vi "UHR-Fleezers Control (host) -Leonardo 04-2018 V4_fish.vi"(0 "Tab Green FB":T5(tab)=enum."Trap Control (RF)") -> ()   [LabVIEW 2014] (continued)
0.042672538888036585, 0.042644759345288163, 0.04261697980253975, 0.04258920025979133, 0.04256142071704291, 0.04253364117429449, 0.04250586163154607, 0.04247808208879765, 0.04245030254604923, 0.04242252300330081, 0.042394743460552387, 0.04236696391780398, 0.04233918437505556, 0.04231140483230714, 0.042283625289558716, 0.042255845746810294, 0.04222806620406188, 0.04220028666131346, 0.04217250711856504, 0.042144727575816616, 0.0421169480330682, 0.04208916849031978, 0.04206138894757136, 0.04203360940482294, 0.04200582986207452, 0.0419780503193261, 0.041950270776577675, 0.04192249123382926, 0.041894711691080846, 0.041866932148332425, 0.041839152605584004, 0.04181137306283558, 0.04178359352008716, 0.04175581397733874, 0.04172803443459032, 0.0417002548918419, 0.04167247534909349, 0.04164469580634507, 0.04161691626359665, 0.04158913672084823, 0.041561357178099806, 0.0415335776353514, 0.04150579809260298, 0.041478018549854556, 0.041450239007106135, 0.041422459464357714, 0.04139467992160929, 0.04136690037886087, 0.04133912083611246, 0.04131134129336403, 0.04128356175061562, 0.04125578220786719, 0.04122800266511878, 0.04120022312237036, 0.04117244357962194, 0.041144664036873516, 0.041116884494125094, 0.04108910495137668, 0.04106132540862826, 0.04103354586587984, 0.041005766323131417, 0.040977986780383, 0.04095020723763458, 0.04092242769488616, 0.04089464815213774, 0.04086686860938932, 0.0408390890666409, 0.04081130952389249, 0.04078352998114407, 0.040755750438395646, 0.040727970895647225, 0.040700191352898804, 0.04067241181015039, 0.040644632267401976, 0.04061685272465355, 0.04058907318190513, 0.04056129363915671, 0.04053351409640829, 0.04050573455365987, 0.04047795501091145, 0.040450175468163034, 0.04042239592541461, 0.0403946163826662, 0.04036683683991778, 0.04033905729716935, 0.040311277754420935, 0.040283498211672514, 0.0402557186689241, 0.04022793912617567, 0.04020015958342725, 0.040172380040678836, 0.04014460049793042, 0.040116820955182, 0.04008904141243358, 0.04006126186968516, 0.04003348232693674, 0.04000570278418832, 0.03997792324143991, 0.03995014369869149, 0.039922364155943066, 0.039894584613194645, 0.03986680507044622, 0.0398390255276978, 0.03981124598494939, 0.03978346644220096, 0.039755686899452546]
  in  "Tab APD Timing":enum32{"Timing", "MCL Scan", "Analog Out"}(tab)=enum."MCL Scan"
  out "APD 2 Gate Late Counter":u32
  out "APD 2 Gate Relative Phase":i16
  in  "Phase Adj. (APD 2 Gate)":i16=20
  in  "Initial Phase Adjustment (APD 2 Gate)":i16=45
  out "APD 1 Gate Late Counter":u32
  in  "- phase (APD 1 Gate)":bool
  in  "+ phase (APD 1 Gate)":bool
  out "APD 1 Gate Relative Phase":i16
  in  "Phase Adj. (APD 1 Gate)":i16=20
  in  "Initial Phase Adjustment (APD 1 Gate)":i16=50
  in  "Save APD Data\nwith Trap Data":bool=TRUE
  out "APD FIFO Elements Remaining":u32
  in  "- phase (APD Acq)":bool
  in  "+ phase (APD Acq)":bool
  out "APD Acq Late Counter":u32
  out "APD Acq Relative Phase":i16
  in  "Phase Adj. (APD Acq)":i16=20
  in  "Initial Phase Adjustment (APD Acq)":i16
  in  "Invert APD Gate":bool caption="Invert Gate"
  in  "APD Gate OFF Count":u32=450 caption="Gate OFF Count"
  in  "APD Gate ON Count":u32=150 caption="Gate ON Count"
  in  "APD Gate":enum32{"ON", "OFF", "Interlace"}(radio)=enum."Interlace"
  in  "APD Integration Time (s)":dbl=0.01 caption="Integration Time (s)"
  out "APD Acq Rate (Hz)":dbl=100.0 caption="Rate (Hz)"
  out "APD Samples/FIFO Acq.":dbl=30.0
  out "APD Elements/DMA read":u32=60
  out "APD Int. Count":u32=400000 format="%.0p"
  in  "+ phase (APD 2 Gate)":bool
  in  "- phase (APD 2 Gate)":bool
  in  "APD FIFO Depth (requires restart)":u32=300000 format="%.0p"
  in  "Tab MCL Misc":enum32{"PSD X", "PSD Y", "Other Data Channel"}(tab)
  out "Data map":dbl[][](graph)=[[-0.01671932143166878, -0.016392818706373227, -0.016060241502617766, -0.016885058281480972, -0.016633639866051188, -0.01614297111485056, -0.01624632439809061, -0.016223291898502697, -0.016322135358181895, -0.015998827366942206, -0.01674383457317074, -0.016349622303473588, -0.01611571290004051, -0.015972334649942688, -0.016306900004507047, -0.016265804263496074, -0.0160006281874421, -0.01579815848604542, -0.015557994770877373, -0.01623934207097493], [-0.016401746716030643, -0.016486228679580477, -0.016405819418185925, -0.017006941359896506, -0.01609698301441303, -0.0159938373980257, -0.015449969664593804, -0.016068061784641922, -0.016115383931390913, -0.015648222289449794, -0.01653040435156989, -0.01664368093936457, -0.015976629115606142, -0.015769041987412753, -0.015716784490458328, -0.016104708313091028, -0.015807740113897233, -0.016007795937736217, -0.015716865824611653, -0.016131560547170874], [-0.016881180243279052, -0.016682362901092443, -0.01653521208533211, -0.016569663649832547, -0.016584350108926265, -0.015788034358096, -0.01572997381191265, -0.016848256863673278, -0.016450971094654886, -0.016646544202256155, -0.016533647976865372, -0.01643411945121718, -0.01642968729491641, -0.015287525792493872, -0.015664412933211656, -0.016705160893495323, -0.01634751515697455, -0.016385950364931786, -0.01641611962972788, -0.016336369365154098], [-0.016944386833653874, -0.017209095062396696, -0.01643647162326984, -0.0169434622427136, -0.01645749558522405, -0.016283892481898044, -0.016603972603686925, -0.016019804038190342, -0.01633990863890397, -0.016779562572954584, -0.01649257003377154, -0.01633196294664365, -0.01681717360495772, -0.016151141680784836, -0.015631110690343758, -0.01616762209708058, -0.01570812545409377, -0.016238042109499973, -0.016140009377557954, -0.015480352129179791], [-0.016627380272623872, -0.016987040432100503, -0.0162998105424607, -0.01635693474229572, -0.016728613514399027, -0.015877063835195653, -0.01632422175035657, -0.015987062444069455, -0.016082210905250194, -0.016795453503208664, -0.0170165982501747, -0.016041147401410074, -0.015844635002206515, -0.01588368721722097, -0.016415515701510675, -0.01625686223052733, -0.015522307984761095, -0.016125254990784654, -0.016133227363549094, -0.016093654313254407], [-0.016918226627058684, -0.016546339201955095, -0.016238630263811032, -0.01698719582491472, -0.016111760237599002, -0.016169388046078873, -0.01635628471807927, -0.016477982760217016, -0.016022494806163096, -0.01635452184408291, -0.016437829589091835, -0.01620151587720066, -0.016192846971583803, -0.016361330735626047, -0.015920360440429684, -0.015596058601637491, -0.015839057608204695, -0.01590683226225114, -0.016147455226815495, -0.016061133185195295], [-0.016634948322751798, -0.016569012123295146, -0.01662465918442623, -0.01677966319575081, -0.016244237674368125, -0.016934028324529424, -0.015994902143504568, -0.01577806108898649, -0.015702882269567658, -0.01637426003303808, -0.016516796952512437, -0.01646180977161214, -0.017050841082784957, -0.015210920961454804, -0.016180578875882937, -0.01607665952058283, -0.01643056573904152, -0.01624726697921726, -0.016811320756287537, -0.015704237088347145], [-0.016797771368752906, -0.01616083928333069, -0.016453251971550422, -0.01638112181272177, -0.01590261356594244, -0.01608147749759244, -0.016020370516697566, -0.01666407664114518, -0.01638481284701757, -0.016175328500489604, -0.015634096607040564, -0.01659680945708638, -0.01626086024191585, -0.016096523812787963, -0.015760521307245458, -0.01615157630765101, -0.01563169067138887, -0.016252628883934674, -0.016238504839935688, -0.016296984466382107], [-0.01667963634531472, -0.015869270181190567, -0.01639782773103042, -0.01636439382881424, -0.01666285543553242, -0.016692875783958446, -0.016121724588237546, -0.016079967645743654, -0.01632967716613466, -0.0165840590606689, -0.01625421166976198, -0.016098422085292646, -0.016839026057991122, -0.01618499247497865, -0.015391600029151147, -0.016339655626827314, -0.015612166346566772, -0.015935379715422582, -0.015751812989013417, -0.016043659821299468], [-0.016548348623009697, -0.016991017407413864, -0.016507403110123067, -0.016536793878207376, -0.016691120016137963, -0.01577327808799238, -0.016241167864690632, -0.016068735698142586, -0.015840387814149363, -0.016134357225980472, -0.015841333026290365, -0.0163038114660657, -0.01664004009343323, -0.015517995684912076, -0.01510255011893393, -0.016011490555515644, -0.01579492187645071, -0.016061693314939115, -0.016070791499276448, -0.015958266458419586], [-0.017158052821315092, -0.016990745992594425, -0.01659770916824297, -0.016038631482428484, -0.016146804022232154, -0.01576224906436341, -0.016188682344964726, -0.016682643876198163, -0.016363274145684666, -0.01639850086318443, -0.015896821220835786, -0.015725853678146523, -0.01601090474694708, -0.015561700057052, -0.015999978841264924, -0.01601836056022779, -0.016765653382201824, -0.016096916088969352, -0.016073837821775124, -0.015692878955540758], [-0.01663419671959083, -0.016709422884628247, -0.017440867448447667, -0.016794212435564802, -0.016747490720603195, -0.017381751349696366, -0.016447004176656708, -0.016200072448833015, -0.016045160782039845, -0.01632124390318996, -0.01679169430451878, -0.016160654157203025, -0.016749084172300182, -0.015317451826774697, -0.01616958983467165, -0.015522373654827837, -0.016042029406509332, -0.016273918604509642, -0.016417636335760946, -0.01644358854973573], [-0.016334373306253872, -0.016757773312361682, -0.016379901767213538, -0.016648254461466998, -0.016415141976627915, -0.016163802224577726, -0.01585938187523836, -0.01585373106879133, -0.015975877635193418, -0.01599748687305492, -0.016737850820893803, -0.01594503246026053, -0.01605934628998727, -0.0158171814426758, -0.015143820145612868, -0.016535815039113604, -0.01611350163485256, -0.01603586147994221, -0.016191023597649318, -0.015673182413705102], [-0.016700857633048308, -0.017051706885756718, -0.016395162126784154, -0.016864165985049667, -0.01667278712452, -0.016023236569300325, -0.015936447644162688, -0.01626053315184134, -0.016666644977778797, -0.01651990276982608, -0.01690611112853018, -0.016570014742366936, -0.016014494913507715, -0.016334286074074115, -0.01621235686701924, -0.01653022812336152, -0.01583634924223019, -0.016281303974484927, -0.01653990312391212, -0.015384206653677268], [-0.016471441301573585, -0.01647096314202187, -0.016715886966535524, -0.015878302888681167, -0.016818970876684446, -0.016713152489800882, -0.0154648252478201, -0.016328530500277577, -0.015836781582585016, -0.01591923201699931, -0.016315094505816256, -0.015951841421804724, -0.01608430179945204, -0.015957272458344565, -0.015751249520465478, -0.016350306857141315, -0.015517909552404317, -0.015884662571158274, -0.016211720964471307, -0.01537858018482844], [-0.01674440523726064, -0.016870567772511377, -0.016213148874409115, -0.016888734754126403, -0.017090609693170035, -0.01659256562080198, -0.01625635717081822, -0.016107107745803876, -0.016234190134722645, -0.016577197956586683, -0.01658670958631228, -0.016563728816596346, -0.016688515093891267, -0.016736196160361996, -0.015994597797780702, -0.016061666241292242, -0.015206770358209283, -0.01656914278587982, -0.01606315534154764, -0.015681866815853374], [-0.016944331036564515, -0.017205260427342613, -0.01677120483170293, -0.016402843466637763, -0.01674116281665193, -0.016423395631415146, -0.01525500299962603, -0.01627542397053335, -0.016664853908603776, -0.01620332976021642, -0.015950564835878013, -0.01610107356411497, -0.016396683154864377, -0.015976631236977498, -0.015478300298060717, -0.015835627632208554, -0.01604600189786053, -0.015850180758366084, -0.01603596051783181, -0.015769623989901102], [-0.016857923835780924, -0.016573198672727902, -0.016660307411618773, -0.016198760579099178, -0.016151481374992453, -0.01623511193332007, -0.015818969815924802, -0.01644510963983431, -0.015972042272190907, -0.01666642359581892, -0.01666443700190194, -0.016438254918363447, -0.016138118663893655, -0.015691974269895034, -0.016587077315345165, -0.015965118060360686, -0.015699839910512218, -0.01561194620613338, -0.016186792034230305, -0.016197922335520733], [-0.016756662992071368, -0.017021980605505502, -0.01671540550240299, -0.016161860765568574, -0.016256637402529132, -0.01604906368842445, -0.016092507257301394, -0.01617438393323743, -0.016105543848009572, -0.016246592326198385, -0.016142744624025374, -0.016159689527728567, -0.016177575339496836, -0.015961391152738445, -0.015789242903564853, -0.016290502978789936, -0.01590902706214275, -0.016035878036151207, -0.0163699057102928, -0.016166856731619543], [-0.016230743921604517, -0.01699457586491366, -0.01691575006710251, -0.01691567874763252, -0.016632348348462205, -0.01564006866069024, -0.015669555325846102, -0.01675726036853814, -0.015659388136628594, -0.01633203630678029, -0.016275904140963263, -0.01599466989252362, -0.01670183436780044, -0.016544315654085533, -0.015882735536646285, -0.01634814491721433, -0.015693511174422668, -0.015857069610244905, -0.015293298228102974, -0.01570879180052374], [-0.016746550537387085, -0.016635756849929545, -0.01704192789682773, -0.01592942336549498, -0.016565335498658518, -0.016559981627150607, -0.016370390094235444, -0.016204117687222342, -0.01636993721064581, -0.016019023809705737, -0.01624713908528634, -0.01653713290533686, -0.01654191191022731, -0.015871787270804183, -0.016600435605206076, -0.016053794928515903, -0.015786397557799592, -0.016167422435048453, -0.016149009764007245, -0.015779827376486453], [-0.017141787830569893, -0.01685604196926299, -0.016770676218784503, -0.01657265724540346, -0.016973351148096293, -0.016347677914333066, -0.015700463473615457, -0.0157292679709582, -0.016282549721629708, -0.015799962485816943, -0.0169651499113691, -0.017005390716294616, -0.01616841590634147, -0.01579805772887789, -0.015884669429112312, -0.01687947774540062, -0.015546104827296667, -0.01606408203496036, -0.015764690031214893, -0.016077969368821936], [-0.01755128513645066, -0.016614441354853425, -0.01642295621649906, -0.016572002735089818, -0.016539344978417192, -0.01665672671509038, -0.01610564101766388, -0.0167710479608722, -0.01604147346071364, -0.015915051759660022, -0.01690954942974296, -0.01618215110656205, -0.01687103577661275, -0.015704550539293104, -0.01567934362211993, -0.015968805810754147, -0.01586985536309292, -0.015848872001954256, -0.015923479964089694, -0.015604572794266433], [-0.01700702905775247, -0.016405242404623068, -0.016957584669743626, -0.01649808356316003, -0.015831866505709048, -0.01650461850371917, -0.015987113078007254, -0.015834023912635466, -0.015505062044615166, -0.016233666617861173, -0.016028249584376462, -0.016292798595496677, -0.016811560188299345, -0.015802581883183398, -0.015195148613460024, -0.015765465657774175, -0.016294889918615045, -0.01647530657977607, -0.016354233471026363, -0.01618598563271133], [-0.016283357847285636, -0.01655641981831666, -0.016127059444156554, -0.016293855360523378, -0.01631947219897442, -0.016398508430939616, -0.0164960599809452, -0.01635229032278839, -0.016150072161158744, -0.01646190473964058, -0.016283962555137702, -0.01689040784367708, -0.016767163139998632, -0.016438000493173108, -0.015954956500429416, -0.016569056147695202, -0.016605504963760735, -0.015329313107534112, -0.01578842030659742, -0.015421959499234628], [-0.016479987599589248, -0.01644678482494596, -0.016512996052180717, -0.01623094473834884, -0.016604746810030113, -0.016230213519226107, -0.016359208382350467, -0.01609761921903255, -0.016464485575532387, -0.015985272322973462, -0.015774520381458212, -0.01632178510310122, -0.016823351362691343, -0.01643553466150876, -0.015434648968053383, -0.01640702032901096, -0.015639626970513753, -0.01608966370811705, -0.016018362361111357, -0.01607982188546427], [-0.016959739645157706, -0.016680901866661726, -0.015836205448559966, -0.016650560318028734, -0.015979362423611275, -0.015641297610719303, -0.015788746501915876, -0.016033508703118756, -0.01595573902096323, -0.016363948579213562, -0.016349864006002027, -0.016495398899173445, -0.016242648234899834, -0.016920033344786076, -0.016276181128461735, -0.016473741446416813, -0.015963577017676644, -0.015565621002678179, -0.01634988477510272, -0.016759987490697584], [-0.016465195958807775, -0.016666490625723715, -0.016658908615375, -0.01597417902764041, -0.016394946754303752, -0.016153528909152313, -0.016275277887248356, -0.016575820504070977, -0.016165440248126276, -0.0158334592734765, -0.016393067206609387, -0.016885479811953534, -0.016471593134372298, -0.017124297138208497, -0.01548599428740715, -0.016309544928836586, -0.015739577267293366, -0.016315386973421362, -0.016361118135948566, -0.016635949477566882], [-0.016680470580762462, -0.016967020008211, -0.017070403001069857, -0.015793158201855152, -0.01661718510493328, -0.01621301409151063, -0.015497330917384148, -0.016267684516616924, -0.015545683307124036, -0.01584462817622427, -0.016830529260392843, -0.016203294725707643, -0.016943290418910587, -0.015581438668509352, -0.015578492450734066, -0.01643368853494311, -0.016285119780950222, -0.015912568651561352, -0.015719368411857025, -0.015732642681635923], [-0.017056323385982973, -0.017071971641855074, -0.01624203196673346, -0.016577086084052214, -0.016198385464505236, -0.015959998936922397, -0.015388246890736087, -0.01690871560472578, -0.016520770777269024, -0.016719342780151844, -0.01589885976225658, -0.016316317143634285, -0.015927259253864068, -0.01613903479860508, -0.015938319643326725, -0.015996730877187566, -0.01552190097834432, -0.016279927776335308, -0.015995176436170485, -0.015804091652970826], [-0.017190435316337342, -0.016575163169333516, -0.01629659819256952, -0.016774256975583077, -0.015978440181354282, -0.016162892801179076, -0.01620143768882657, -0.016215940324925678, -0.016085616640623322, -0.01624795446292185, -0.015590279490139558, -0.016351775677783426, -0.01628162630120476, -0.016736583715483217, -0.015290607493835316, -0.01675006130238602, -0.016112399997689694, -0.016085396155956493, -0.01584495781031281, -0.016031709625742012], [-0.017226310157841672, -0.0164663033859778, -0.01638852606295136, -0.01642215259901681, -0.016566243818266997, -0.016484045986143257, -0.016452209817223822, -0.016464707609223313, -0.01598467645947642, -0.016476401570535384, -0.015529223129381136, -0.016802343788985992, -0.016417294815804, -0.016305476633183012, -0.015407470515554668, -0.01588918182788552, -0.015839354895906106, -0.016859219988342257, -0.016188952756112908, -0.015382351679335257], [-0.017044276140355946, -0.016525294382434108, -0.01600036800318285, -0.01692841042125611, -0.016063543400203904, -0.0167008216867912, -0.01583944304325613, -0.015982843969462788, -0.01610446772754332, -0.01650934416727942, -0.016660683575282727, -0.016326108469991264, -0.01614299940648814, -0.016050548764700443, -0.016131072933532012, -0.016315196635999143, -0.016225473554238007, -0.01551847935196565, -0.015874550726858914, -0.01566897000262655], [-0.016174756903461544, -0.01692999553661901, -0.01705167048362926, -0.01660949009366751, -0.016107419352032235, -0.016188509519945497, -0.015585853922651487, -0.01612262091090234, -0.016426426055949322, -0.01609822137272688, -0.016735004284984756, -0.016043599908818165, -0.016651804571551146, -0.01556136051538674, -0.015408827232157843, -0.015855874683892428, -0.015887023972496795, -0.01599811437353065, -0.015655637769778918, -0.015893480415302176], [-0.016396467105890343, -0.01690556505247584, -0.0163054855200399, -0.016446662941364928, -0.01622691165873451, -0.016690239637868323, -0.015785441074554568, -0.016620593981308673, -0.015765446409343138, -0.016270811628848948, -0.016094841434208293, -0.01632812303243944, -0.01619217328151394, -0.015836234359203484, -0.016074598803568225, -0.01532030760600064, -0.01657169575010852, -0.016393493124135967, -0.01597552762388542, -0.015565046037824628], [-0.016299520764774443, -0.016637551393085426, -0.016299287907039765, -0.01610813956937386, -0.016305200311999217, -0.016601228593523636, -0.016288899767132464, -0.016305235511310533, -0.016063090550620947, -0.01683118193989227, -0.015518909238992087, -0.01620458965118359, -0.01645647074542291, -0.015677575909554008, -0.015332584749786342, -0.016079840062543812, -0.016278322310175185, -0.01605786016548567, -0.01657700147769983, -0.01606751816440997], [-0.016441387384698882, -0.017325914631361444, -0.017225293509456174, -0.016118796157285526, -0.016362377734664042, -0.01516634537172325, -0.01608508664570788, -0.01572299536201756, -0.01616493137153105, -0.01621315960010322, -0.016750280429064943, -0.016228195768808316, -0.01653543568323192, -0.01645026349483051, -0.016050647149129828, -0.01642593239180811, -0.0161192309302286, -0.01629438826737352, -0.015557310160813994, -0.016021567325025916], [-0.01686693458295582, -0.016740786564424494, -0.01648453245605215, -0.01640092243822592, -0.01555424864442638, -0.01667099748425638, -0.016069415470156286, -0.01638225749592203, -0.01607630099787768, -0.01614344420814296, -0.016216929728619375, -0.016309670684273796, -0.015741358140653132, -0.015770999475234804, -0.01601963602183988, -0.01615265943136728, -0.016152653946118384, -0.01698528285009184, -0.015969420465915152, -0.01578449323306024], [-0.01598619419452168, -0.016362732490235912, -0.016433844312774552, -0.016357999277320685, -0.015969441982301692, -0.01621147526376268, -0.016085473373391473, -0.016306341052304336, -0.015855664982231947, -0.015900633884010838, -0.016902356755211914, -0.016434765274207237, -0.016180164153866673, -0.015973977144992546, -0.01589274164800459, -0.01640268056199417, -0.016415161422386984, -0.01617112040367598, -0.016354725082739732, -0.016206639631885546], [-0.016048964224847716, -0.016745007333129024, -0.017180534108641177, -0.016329775174222558, -0.016582289070660373, -0.016075138720435006, -0.016345162602564738, -0.016090296577092385, -0.016153752753705675, -0.016379459268123033, -0.016228628993078524, -0.016712275509199688, -0.015795168051192618, -0.015386431874568587, -0.01610093851445945, -0.01633598707495066, -0.015921284689633122, -0.016330315102764423, -0.015994974665173196, -0.015537812293197398]]
  in  "Channel":i32=4
  in  "Abort MCL Scan":bool
  out "MCL Scan I":u64=2
  out "MCL Scanning":bool
  in  "Start MCL Scan":bool
  out "wait to reset values":bool
  in  "Tab MCL Scan Settings":enum32{"Scan Settings", "MCL FPGA Loop Timing"}(tab)
  out "Total Time (s)":dbl=48.0
  in  "Scan lines (y)":u64=20
  in  "Fast Scan Dir":bool=TRUE
  in  "2D or 1D Scan":bool=TRUE
  out "Initial X":dbl=1.6310662274449115
  out "Initial Y":dbl=2.5691326639606933
  out "Time/f+b scan (s) (MCL)":dbl=2.4 caption="Time/scan (s)"
  in  "Number of scans (MCL)":u64=1 caption="Scans"
  in  "Scan steps (MCL)":u64=40 caption="Scan steps (x)"
  in  "N APD Samp/step":dbl=3.0
  in  "Scan Range (V)\n(of steps)":dbl=3.5
  in  "Restart DMA? (MCL)":bool=TRUE caption="Restart DMA?"
  in  "Continuous MCL Scanning":bool caption="Cont. Scanning"
  in  "Center Scan":bool=TRUE
  in  "Save Data (MCL)":bool=TRUE caption="Save Data"
  out "Actual Incr. int (MCL)":i16=462 caption="Incr. int"
  out "Desired incr (int)":dbl=462.098717948718
  out "Desired Scan Incr (V)":dbl=0.14102564102564102
  out "N sets should be saved (MCL)":dbl=160.0 caption="N sets should be saved"
  out "Data points/scans (MCL)":dbl=4800.0 caption="Data points/scans"
  out "Data points/scan (f+b)":dbl=240.0 caption="points/scan (f+b)"
  out "Cycles/step (MCL)":u64=2000 caption="Cycles/step" format="%.0p"
  out "Actual MCL Inc (V)":dbl=0.14099551377910702
  in  "Phase adjust (MCL)":i16 caption="Phase adjust"
  out "Relative Phase (MCL)":i16 caption="Relative Phase"
  in  "Initial Phase Adj. (MCL)":i16 caption="Initial Phase Adj."
  in  "Update Count (MCL)":u32=600
  in  "+ phase (MCL)":bool
  in  "- phase (MCL)":bool
  out "MCL Late Counter":u32
  in  "APD 1 AO Mult.":i16=1 min=1
  in  "APD 2 AO Mult.":i16=1 min=1
  in  "Tab Control 7":enum32{"Green FB Signals", "Slow MCL Scan"}(tab)
  out "Green FB Plot":dbl(graph)=-10.00030518509476
  out "MCL Scan 2":cluster{"Begin (V)":dbl, dbl, dbl[]}(graph)
  out "MCL Scan":cluster{"Begin (V)":dbl, dbl, dbl[]}(graph)
  in  "GI Frequency, ON count":u32=150 min=1 step=1
  in  "Invert GI":bool
  out "GI Late Counter":u32
  in  "Phase adj. (GI)":i16=5
  out "GI relative phase":i16
  in  "+ phase (GI)":bool
  in  "Initial Phase Adjustment (GI)":i16=4
  in  "GI Frequency, OFF count":u32=450 min=1 step=1
  in  "- phase (GI)":bool
  out "Green FB Signals (V)":cluster{"Y":dbl, "X":dbl, "Sum":dbl}={"Y"=-0.999969482421875, "X"=1.0, "Sum"=-10.00030518509476}
  out "Relative phase (Green FB)":i16
  in  "+ phase (Green FB)":bool
  in  "- phase (Green FB)":bool
  in  "Green FB Count":u32=600
  in  "Phase adj. (Green FB)":i16=10
  in  "Initial Phase Adjustment (Green FB)":i16=50
  in  "Green FB On/Off":bool
  in  "Green int current ON count adj":u32=150
  in  "Green FB Gains":T10={"proportional gain (Kc)"=10, "integral gain (Kc*Ts/Ti)"=5, "derivative gain (Kc*Td/Ts)"=0}
  in  "Green FB Setpoint (mV)":dbl=100.0
  in  "- phase (GI) 2":bool
  in  "Initial Phase Adjustment (GI) 2":i16=-100
  in  "+ phase (GI) 2":bool
  out "GI relative phase 2":i16
  in  "Phase adj. (GI) 2":i16=20
  out "GI Late Counter 2":u32
  in  "Negate X signals":bool
  in  "Trap Position FIFO Depth":u32=300000 format="%.0p"
  in  "# Samples/trap":u32=20000 format="%.0p"
  out "Trap AI Elements/DMA read":u32=320000 format="%.0p"
  out "Ave. Rate (Hz)":dbl=200000.0 format="%#_6p"
  out "Trap AI FIFO El. Rem.":u32 format="%.0p"
  in  "Phase adj. (AI1)":i16
  out "Relative phase (AI1)":i16
  in  "+ phase (AI1)":bool
  in  "- phase (AI1)":bool
  out "Late Counter (AI1)":u32
  in  "Initial Phase Adjustment (AI1)":i16=185
  out "AI rate (Hz)":dbl=200000.0 format="%#_6p"
  in  "AI Count (ticks)":u32=200
  out "# Samples/channel":u32=40000 format="%.0p"
  in  "Trap AI FIFO Depth":u32=340000 format="%.0p"
  in  "Detector Type":string(combo)="UCB Fleezers 052511"
  in  "N Acq Sets (Traps + Fl.)":i16=3
  in  "Sets to FIFO (Traps)":T15={"Set 1"=TRUE, "Set 2"=TRUE, "Set 3"=FALSE}
  in  "FPGA Ave.":dbl=1.0 min=1.0 step=1.0
  out "Ave. Period (s)":dbl=5e-06 format="%#_6p"
  out "DMA Update Period (s)":dbl=0.3
  out "FPGA Averaging":bool
  out "Trap Sets":u32=2
  out "Counts/DMA":dbl=12000000.0 format="%#_6p"
  out "Trap Pos FIFO El Remaining":u32=171
  out "Trap Pos Elements/DMA read":u32=120000 format="%.0p"
  out "Trap AI FIFO Timeout":u16
  out "Trap Pos FIFO Timeout":u16
  out "Waveform Chart":i32(graph)=320000
  out "error out 2":errorcluster
  in  "Lost Tether Alarm Threshold (pN)":dbl=0.5
  in  "AOM X Cal (nm/MHz)":dbl=160.0
  in  "MCL X Cal (nm/V)":dbl=1174.0
  out "X RF Amplitude Limits (%)":T16={"Minimum"=0.0, "Maximum"=75.0, "Increment"=1.0}
  out "X RF Frequency Limits (MHz)":T16={"Minimum"=60.0, "Maximum"=90.0, "Increment"=1.0}
  out "Y RF Frequency Limits (MHz)":T16={"Minimum"=60.0, "Maximum"=90.0, "Increment"=1.0}
  out "Y RF Amplitude Limits (%)":T16={"Minimum"=0.0, "Maximum"=75.0, "Increment"=1.0}
  in  "Manip. X?":bool=TRUE
  in  "Manip. Y?":bool
  in  "Force Manip Abort":bool
  out "Read cal error":errorcluster
  in  "DAQ Delay (ms)":u32=1000
  in  "Start Scan":bool
  in  "Scan axis":bool
  in  "Osc. amp. (V)":dbl=5.0
  in  "Osc. center (V)":dbl=5.0
  in  "Osc. freq. (Hz) 2":dbl=1.0
  in  "MCL Mode":u16(ring) items=["Manual Positioning", "Sinusoidal Wave", "Linear Scan"]
  in  "Begin (V)":dbl
  in  "End (V)":dbl=10.0
  in  "N Points":dbl=20.0
  in  "Delay to Interlace (s)":dbl
  in  "Delayed Interlace Start":bool
  in  "Read Lateness and Rel Phase":bool
  out "Vec Mean of T1 T2":dbl[](array[numeric])=[1.039290883164312, 1.038787885614062]
  in  "Cal read wait (s)":u32=5
  out "Time tether formed":timestamp=timestamp(3371146929.513132 s since 1904-01-01)
  in  "Chemyx Syringe Pump Serial Port":refnum<visa-resource-name>="ASRL3::INSTR"
  in  "Limit Min (MHz)":dbl=10.0 caption="Min (MHz)"
  in  "Limit Max (MHz)":dbl=16.0 caption="Max (MHz)"
  in  "Limits Enable":bool=TRUE caption="Enable"
  out "AI labels":string[](array[string])=["T1 Y", "T1 X", "T1 Sum", "T2 Y", "T2 X", "T2 Sum", "T1 FB X", "T2 FB Sum", "T2 FB X", "T2 FB Sum", "PSD Y", "PSD X", "PSD Sum"]
  in  "Save Trap Pos. Data":bool=TRUE
  in  "ESP Port":refnum<visa-resource-name>="COM4"
  in  "Axis 3":string="0.00500\r\n"
  in  "Axis 2":string="0.00500\r\n"
  in  "Axis 1":string="0.00500\r\n"
  in  "Axis 3":string="0.20000\r\n"
  in  "Axis 2":string="0.20000\r\n"
  in  "Axis 1":string="0.20000\r\n"
  in  "Activate Joystick":bool
  in  "ESP ZL-Limit":string="-0.09900"
  in  "ESP ZR-Limit":string="0.09900"
  in  "error in":errorcluster
  out "error out":errorcluster
  out "Current MCL (V)":dbl=5.657514378627918
  in  "Tracking factor":dbl=-0.45
  out "Zero T1 position":dbl=70.0
  out "Zero MCL x position":dbl=5.6547922360429315
  # "Trap interlacing RF phase control\n\n0 = no phase control\n1 = offset increments each trap cycle by values below\n2 = offset increment increases by increment factor each cycle\n3 = random phase (no parameters set)"
  # "Save Positions of Cambers"
  # "After"
  # "During"
  # "Trap On?"
  # "BD Flow ON?"
  # "Samp Flow ON?"
  # "1"
  # "2"
  # "Trap Display:"
  # "APD Display:"
  # "originally 10k"
  # "Data Saving"
  # "Trap Manipulation"
  # "DAQ"
  # "Central frequency 80 MHz"
  # "INS"
  # "DEL"
  # "Bead Calibration"
  # "Current Location"
  # "Select the chamber to go to"
  # "F4"
  # "Press F12 to move stage\nwith the mouse. F12 to cancel."
  # "F5"
  # "F6"
  # "F7"
  # "F8"
  # "Harvard Pump\n(sample channel for flow exp)"
  # "Chemyx Pump 2"
  # "Units: \n1 = ml/m\n2 = ml/h\n3 = ul/m\n4 = ul/h"
  # "Rate param is ul/h\nVolume param is ul"
  # "Oscillate Set 2 freq. (debugging)"
  # "BD 1"
  # "BD 2"
  # "X"
  # "Y"
  # "AOD Raster Scan"
  # "Approx. trap separations"
  # "X"
  # "Y"
  # "DON'T TURN ON\nUNTIL YOU CLOSE\nTHE LOOP"
  # "FPGA\nreading"
  # "DMA\ntransfer"
  # "APD Gates"
  # "APD 2"
  # "APD 1"
  # "X"
  # "2D"
  # "Y"
  # "1D"
  # "Green FB Measurement"
  # "Green Laser Interlacing"
  # "Digital Gate"
  # "Current Analog Control"
  # "was 87"
  # "originally 600k"
  # "Total AI Rates (NOT rates/trap)"
  # "originally 20k"
  # "(Samples/trap x Trap Sets)"
  # "(Samples/channel x\n8 if averaging (8 channels)\n4 if no averaging)"
  # "Trap 1"
  # "Trap 2"
  # "Flour./Trap 3"
  # "External Video Window"
  # "MCL Position Debugging"
  # "Temporary Control Storage\n(these used to be somewhere else, still want to keep them)"
  # "Y"
  # "X"
  # "Trap Position Difference Limits"
  # "Joystick Control"
  # "Setting Limit for the z-axis"
  # "Errors detected in determing Current Location"
  # "High Jog Velocity"
  # "Low Jog Velocity"
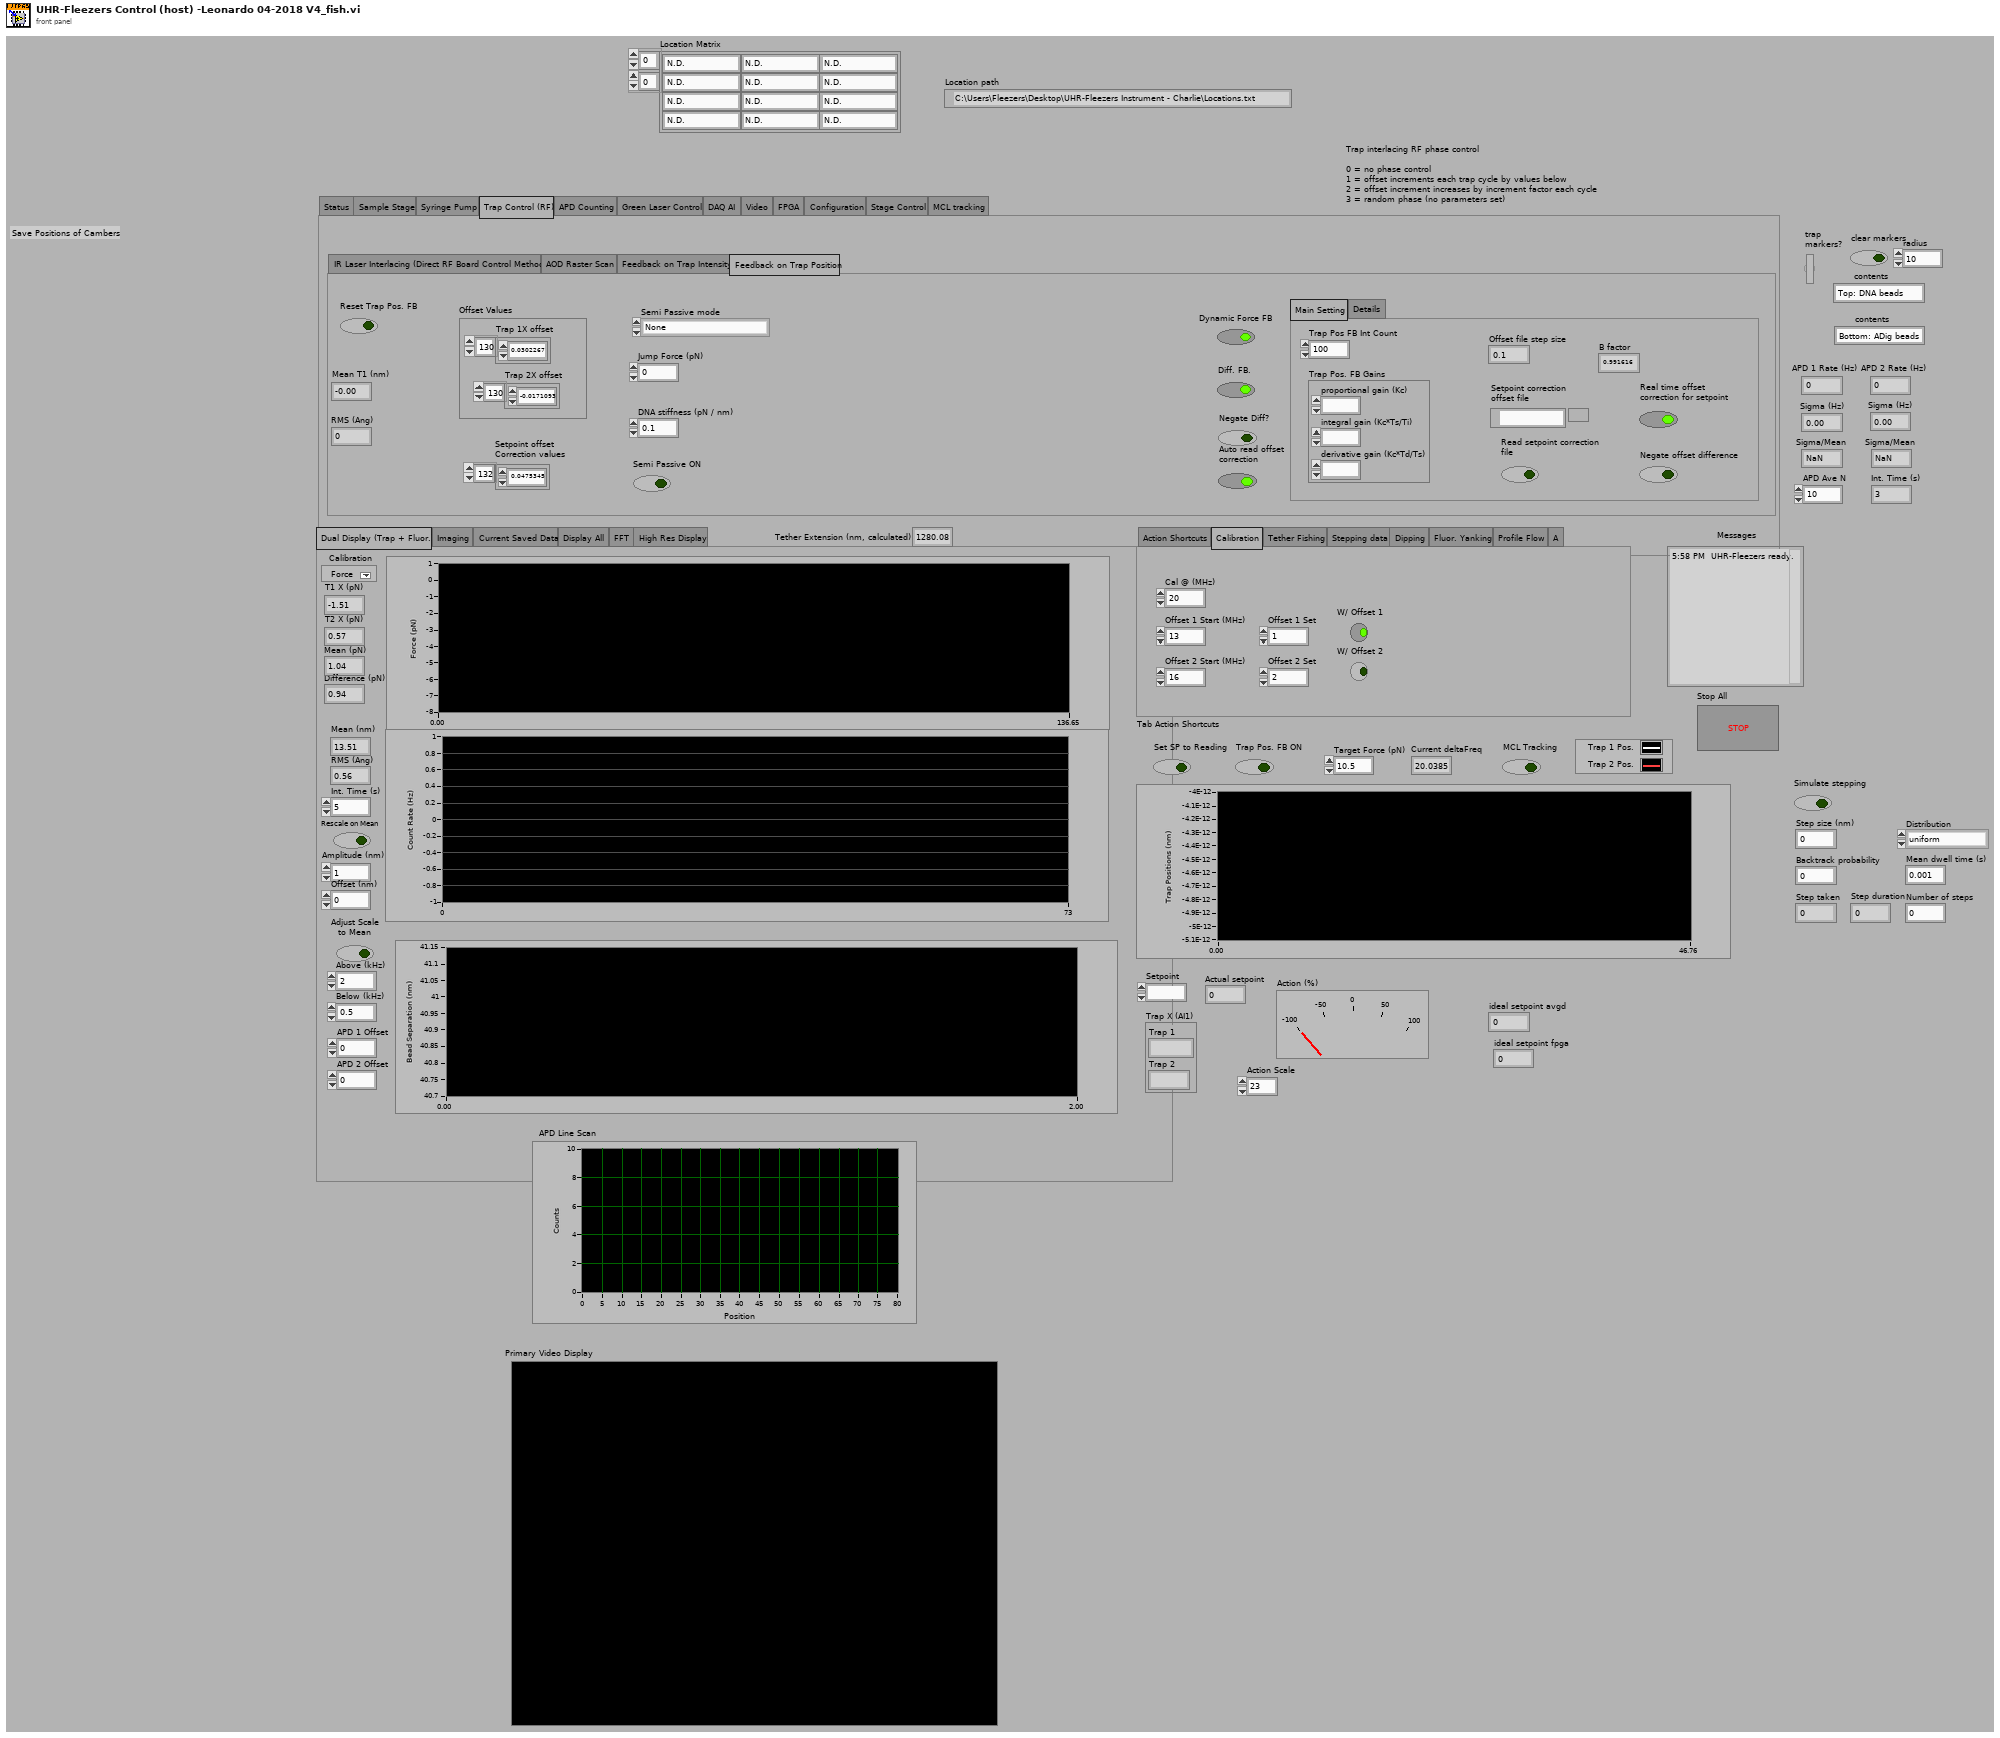
[diagram p1: front panel]
types:
  T1 = cluster{"Trap 1":fxp<+/-,16,1>, "Trap 2":fxp<+/-,16,1>}
  T2 = enum32{"Action Shortcuts", "Calibration", "Tether Fishing", "Stepping data", "Dipping", "Fluor. Yanking", "Profile Flow", "A"}
  T3 = typedef "IMAQ Image.ctl" = refnum<image>
  T4 = enum32{"Dual Display (Trap + Fluor.)", "Imaging", "Current Saved Data", "Display All", "FFT", "High Res Display"}
  T5 = enum32{"Status", "Sample Stage", "Syringe Pump", "Trap Control (RF)", "APD Counting", "Green Laser Control", "DAQ AI", "Video", "FPGA", "Configuration", "Stage Control", "MCL tracking"}
  T6 = cluster{"Pump 1":cluster{"Diameter (mm)":dbl, "Units":dbl, "Volume":dbl, "Rate":dbl}, "Pump 2":cluster{"Diameter (mm)":dbl, "Units":dbl, "Volume":dbl, "Rate":dbl}, "Pump 3":cluster{"Diameter (mm)":dbl, "Units":dbl, "Volume":dbl, "Rate":dbl}}
  T7 = enum32{"IR Laser Interlacing (Direct RF Board Control Method)", "AOD Raster Scan", "Feedback on Trap Intensity", "Feedback on Trap Position"}
  T8 = typedef "LVPoint32TypeDef.ctl" = cluster{"Horizontal":i32, "Vertical":i32}
  T9 = cluster{"Scan Range AOD (nm) 2":dbl, "Step Size AOD (nm) 2":dbl, "Scan Speed AOD (nm/s) 2":dbl, "Number of scans (AOD) 2":u16, "Label":string}[]
  T10 = cluster{"proportional gain (Kc)":i16, "integral gain (Kc*Ts/Ti)":i16, "derivative gain (Kc*Td/Ts)":i16}
  T11 = cluster{"proportional gain (Kc)":fxp<+/-,16,8>, "integral gain (Kc*Ts/Ti)":fxp<+/-,16,8>, "derivative gain (Kc*Td/Ts)":fxp<+/-,16,8>}
  T12 = cluster{"output high":fxp<+/-,16,1>, "output low":fxp<+/-,16,1>}
  T13 = cluster{"Set 1":fxp<+/-,16,1>, "Set 2":fxp<+/-,16,1>}
  T14 = cluster{"Trap 1X offset":dbl[], "Trap 2X offset":dbl[]}
  T15 = cluster{"Set 1":bool, "Set 2":bool, "Set 3":bool}
  T16 = typedef "LVMinMaxIncTypeDef.ctl" = cluster{"Minimum":dbl, "Maximum":dbl, "Increment":dbl}
  T17 = typedef "Image Type" = u32
  T18 = typedef "nirio_resource_hc.ctl" = tag
  T19 = typedef "openfpgaref.initrf.ctl" = refnum<k20>
  T20 = typedef "openfpgaref.8.6.ctl" = refnum<k20>
  T21 = enum16{"CONNECT", "INITIALIZE VALVES", "DISCONNECT", "MOVE VALVE"}
  T22 = cluster{"New Image":T3, "New Image":T3, "New Image":T3, "New Image":T3}
  T23 = cluster{"Location Matrix[0]":string, "Location Matrix[1]":string, "Location Matrix[2]":string}
  T24 = enum16{"open", "replace", "create", "open or create", "replace or create", "replace or create with confirmation"}
  T25 = typedef "XDNodeRunTimeDep.lvlib/timing_clust.ctl" = cluster{"Expected End [f-1]":u64, "Actual End [f-1]":u64, "Finished Late? [f-1]":bool, "Expected End [i-1]":u64, "Actual End [i-1]":u64, "Finished Late? [i-1]":bool, "Expected Start [i]":u64, "Actual Start [i]":u64, "Expected Start [f]":u64, "Actual Start [f]":u64, "Source Name":string, "Structure Name":string, "Period":i64, "Deadline":i64, "Offset":i64, "Start":i64, "Priority":i32, "Timeout":i32, "Mode":T26, "Wakeup Reason":T27, "Error":errorcluster, "Source Type":string, "Secondary Source Type":string, "Global End Time":u64, "Global Start Time":u64, "Frame Duration":u64, "Iteration Duration":u64, "Assigned CPU":i32, "I/O Scan Engine Mode":u32}
  T26 = typedef "XDNodeRunTimeDep.lvlib/nitl_modes.ctl" = enum32{"No Change", "Process missed periods, maintain original phase", "Discard missed periods, maintain original phase", "Process missed periods, ignore original phase", "Discard missed periods, ignore original phase"}
  T27 = typedef "XDNodeRunTimeDep.lvlib/wakeup.ctl" = enum32{"Normal", "Aborted", "Asynchronous wakeup", "Timing source error", "Timed loop error", "Timeout"}
  T28 = cluster{"[0]":i32, "[1]":i32, "[2]":i32, "[3]":i32}
  T29 = cluster{"[0]":i32, "[1]":i32, "[2]":i32, "[3]":i32}[]
  T30 = enum16{"big-endian, network order", "native, host order", "little-endian"}
  T31 = cluster{"Scan Range AOD (nm) 2":dbl, "Step Size AOD (nm) 2":dbl, "Scan Speed AOD (nm/s) 2":dbl, "Number of scans (AOD) 2":u16, "Label":string}
  T32 = cluster{"[0]":dbl, "[1]":dbl, "[2]":dbl, "[3]":dbl, "[4]":dbl, "[5]":dbl}
  T33 = cluster{"Diameter (mm)":dbl, "Units":dbl, "Volume":dbl, "Rate":dbl}
  T34 = cluster{"Left":void, "Top":void, "Width":void, "Height":void}
  T35 = cluster{cluster{"Left":void, "Top":void, "Width":void, "Height":void}}[]
  T36 = enum32{"Normal Display", "Dual Display (APD)", "FFT", "High Res Display"}
  T37 = cluster{"Origin Pixel":cluster{"X":sgl, "Y":sgl}, "Angle Relative to Horizontal (deg)":sgl, "Axis Reference":u32}
  T38 = typedef "Simple Grid Descriptor" = cluster{"X Step":sgl, "Y Step":sgl, "Unit":T39}
  T39 = typedef "Image Unit" = enum32{"Undefined", "Angström", "Micrometer", "Millimeter", "Centimeter", "Meter", "Kilometer", "Microinch", "Inch", "Feet", "Nautical miles", "Standard miles", "Steps"}
  T40 = cluster{"averaging mode":u16, "weighting mode":u16, "number of averages":u32}
  T41 = cluster{"dB On (F)":bool, "unwrap phase (F)":bool, "convert to degree (F)":bool}
  T42 = cluster{string, string, string, string, string, string, string, string}
  T43 = cluster{string, string, string, string, string, string, string, string, string, string, string, string}
  T44 = cluster{string, string, string, string, string, string, string, string, string, string, string, string, string}
  T45 = cluster{string, string, string, string, string, string, string, string, string, string, string, string, string, string}
  T46 = cluster{"BD 1 Frequency 1 (MHz)":dbl, "BD 1 Frequency 2 (MHz)":dbl}
  T47 = cluster{"f0":dbl, "df":dbl, "magnitude":dbl[]}[][]
  T48 = cluster{"Green FB Ch 0":i16, "Green FB Ch 1":i16, "Green FB Ch 2":i16}
  T49 = cluster{"Green FB Ch 0":dbl, "Green FB Ch 1":dbl, "Green FB Ch 2":dbl}
diagram:
  w1 = u16 0 items=["Off", "Approach", "Wiggle", "Extend", "Tether Found"] ("Fish Status")
  w34 = 48
  w37 = 1000000.0
  w99 = T17 2 items=["Grayscale (U8)", "Grayscale (I16)", "Grayscale (SGL)", "Complex (CSG)", "RGB (U32)", "HSL (U32)", "RGB (U64)", "Grayscale (U16)"] ("Image Type")
  w228 = 10.0 ("y")
  w227 = 32767.0 ("y")
  w243 = 6.0  # clock mult.
  w244 = 49152000.0  # TCXO frequ.
  # "Initialize location matrix"
  n1 = flat-sequence {
    tunnel: [w278] -> w21
    tunnel: [w286] -> w154
    tunnel: [w287] -> w173
    tunnel: w21 -> [w293]
    frame #0 {
      w278 = T18 "RIO0" ("resource name")
      n2 = xnode "Open FPGA VI Reference"("resource name"=w278) -> ("FPGA VI Reference Out"=w285:T19)  [unwired: 1 in, 1 out]
      n3 = xnode "Invoke Method"("FPGA VI Reference In"=w285) -> ("FPGA VI Reference Out"=w284:T19, "error out"=w283:errorcluster)  [unwired: 1 in]
      n4 = xnode "Invoke Method"("FPGA VI Reference In"=w284, "error in"=w283) -> ("FPGA VI Reference Out"=w281:T19, "error out"=w282:errorcluster)  [unwired: 1 in]
      n5 = call "Initialize RF boards - with FPGA init only vi v1.vi"("error in"=w282, "FPGA Interface"=w281) -> ("error out"=w279:errorcluster, "FPGA Interface 2"=w280:T19)
      n6 = xnode "Close FPGA VI Reference"("FPGA VI Reference In"=w280, "error in"=w279) -> ()  [unwired: 1 out]
    }
    frame #1 {
      w288 = TRUE
      n7 = xnode "Open FPGA VI Reference"("resource name"=w293) -> ("FPGA VI Reference Out"=w292:T20, "error out"=w291:errorcluster)  [unwired: 1 in]
      n8 = xnode "Invoke Method"("FPGA VI Reference In"=w292, "error in"=w291) -> ("FPGA VI Reference Out"=w290:T20, "error out"=w289:errorcluster)
      n9 = xnode "Read/Write Control"("FPGA VI Reference In"=w290, "error in"=w289, "PMODE"=w288, "RD"=w288) -> ("FPGA VI Reference Out"=w286:T20, "error out"=w287:errorcluster)
      "FPGA error out" <- w287
    }
  }
  n10 = Build Array("DIO count 1 (ticks)", "DIO count 2 (ticks)", "DIO count 3 (ticks)") -> (w145:u32[])
  n11 = Multiply(x="APD Integration Time (s)", y=40000000.0) -> (x*y=w162:dbl)
  n12 = Reciprocal(x="APD Integration Time (s)") -> (1/x=w159:dbl)
  n13 = local write "APD Acq Rate (Hz)"(w159) -> ()
  n14 = local read "AO1"() -> (w222:dbl)
  n15 = local read "AO2"() -> (w221:dbl)
  n16 = local read "Dynamic Force FB"() -> (w23:bool)
  n17 = local read "Negate Diff?"() -> (w22:bool)
  n18 = To Unsigned Long Integer(number=w162) -> (unsigned 32bit integer=w161:u32)
  "APD Int. Count" <- w161
  n19 = local read "Diff. FB."() -> (w24:bool)
  n20 = local read "Scan Increment (MHz)"() -> (w239:dbl)
  n21 = local read "Continuous MCL Scanning"() -> (w209:bool)
  n22 = local read "Fast Scan Dir"() -> (w208:bool)
  n23 = local read "Trap Intensity\nSetpoints (V)"() -> (w254:cluster{"Set 1":dbl, "Set 2":dbl})
  n24 = local read "Number of scans (MCL)"() -> (w210:u64)
  n25 = Multiply(x=w222, y=w227) -> (x*y=w224:dbl)
  n26 = Multiply(x=w221, y=w227) -> (x*y=w226:dbl)
  n27 = Divide(x=w224, y=w228) -> (x/y=w223:dbl)
  n28 = Divide(x=w226, y=w228) -> (x/y=w225:dbl)
  n29 = To Word Integer(number=w223) -> (16bit integer=w220:i16)
  n30 = To Word Integer(number=w225) -> (16bit integer=w219:i16)
  n31 = Not(x=w208) -> (.not. x?=w203:bool)
  n32 = local read "Cycles/step (MCL)"() -> (w211:u64)
  n33 = Multiply(x=w239, y=1000.0) -> (x*y=w246:dbl)
  n34 = local read "Scan steps (MCL)"() -> (w212:u64)
  n35 = local write "Trap Pos FIFO Timeout"(u16 0 ("Trap Pos FIFO Timeout")) -> ()
  n36 = local read "Desired Scan Incr (V)"() -> (w214:dbl)
  n37 = Scale By Power Of 2(n=48, x=w246) -> (x*2^n=w247:dbl)
  n38 = local read "Sets to FIFO (Traps)"() -> (w20:T15)
  n39 = Multiply(x=w244, y=w243) -> (x*y=w242:dbl)
  n40 = Divide(x=w247, y=w242) -> (x/y=w241:dbl)
  n41 = local read "Number Interlace Sets"() -> (w138:u8)
  n42 = Split 1D Array(array=w145, index=w138) -> (first subarray=w147:u32[])  [unwired: 1 out]
  n43 = Add Array Elements(numeric array=w147) -> (sum=w146:u32)
  n44 = property on="AI Count (ticks)" class="DigNum (strict)"("Val(Sgnl)"="AI Count (ticks)") -> ()  [unwired: 2 in, 2 out]
  n45 = local read "# Samples/channel"() -> (w231:u32)
  n46 = local read "Number of F/B Scans (AOD)"() -> (w232:u16)
  n47 = To Quad Integer(1:w241) -> (0:w238:i64)
  n48 = local read "Not-Interlacing Set"() -> (w137:enum32{"Set 1", "Set 2", "Set 3"})
  n49 = To Unsigned Byte Integer(number=w137) -> (unsigned 8bit integer=w143:u8)
  n50 = Index Array(array=w145, index=w143) -> (element=w144:u32)
  n51 = local read "Feedback On/Off"() -> (w257:cluster{"Set 1":bool, "Set 2":bool})
  n52 = Divide(x=40000000.0, y="AI Count (ticks)") -> (x/y=w200:dbl)
  n53 = Multiply(x=w214, y=32767.0) -> (x*y=w216:dbl)
  n54 = local read "Scan steps (AOD)"() -> (w237:u64)
  n55 = local read "All FB On/Off"() -> (w258:bool)
  n56 = local read "Cycles/step (AOD)"() -> (w236:u64)
  n57 = local write "AI rate (Hz)"(w200) -> ()
  n58 = Divide(x=w216, y=10.0) -> (x/y=w215:dbl)
  n59 = Multiply(x=w237, y=w236) -> (x*y=w235:u64)
  n60 = Multiply(x=3276.7, y=w254) -> (x*y=w253:cluster{"Set 1":dbl, "Set 2":dbl})
  n61 = To Word Integer(number=w215) -> (16bit integer=w213:i16)
  n62 = Multiply(x=w235, y=u64 2) -> (x*y=w233:u64)
  n63 = Divide(x=w200, y="FPGA Ave.") -> (x/y=w201:dbl)
  n64 = To Word Integer(number=w253) -> (16bit integer=w252:cluster{"Set 1":i16, "Set 2":i16})
  n65 = Multiply(x=w233, y=w232) -> (x*y=w230:u64)
  n66 = local write "Ave. Rate (Hz)"(w201) -> ()
  n67 = Divide(x=w230, y=w231) -> (x/y=w229:dbl)
  n68 = Unbundle By Name(w20) -> ("Set 1"=w19:bool, "Set 2"=w18:bool, "Set 3"=w17:bool)
  n69 = Unbundle By Name(w252) -> ("Set 1"=w251:i16, "Set 2"=w250:i16)
  n70 = local read "2D or 1D Scan"() -> (w156:bool)
  n71 = local write "Data points/scans"(w230) -> ()
  n72 = local read "Scan BD"() -> (w248:bool)
  n73 = And(x=w257, y=w258) -> (x .and. y?=w256:cluster{"Set 1":bool, "Set 2":bool})
  n74 = local write "Data points/scan (f/b)"(w233) -> ()
  n75 = Reciprocal(x=w201) -> (1/x=w202:dbl)
  n76 = local read "N Acq Sets (Traps + Fl.)"() -> (w193:i16)
  n77 = local write "N sets should be saved"(w229) -> ()
  n78 = Unbundle By Name(w256) -> ("Set 1"=w260:bool, "Set 2"=w259:bool)
  n79 = local read "Interlace"() -> (w139:bool)
  n80 = Select(t=w146, s=w139, f=w144) -> (s? t:f=w136:u32)
  n81 = local write "Update Count (MCL)"(w136) -> ()
  n82 = local write "Total Counts (ticks)"(w136) -> ()
  n83 = local write "Ave. Period (s)"(w202) -> ()
  n84 = property on="2D or 1D Scan" class="Bool (strict)"("Val(Sgnl)"=w156) -> ()  [unwired: 2 in, 2 out]
